vi "LLA_2_ECEF(SubVI).vi"(6 "f":dbl, 9 "alt(i) [m]":dbl, 10 "latd(i)":dbl, 11 "lon(i)":dbl) -> (3 "position":dbl[](array[numeric]))   [LabVIEW 2017]
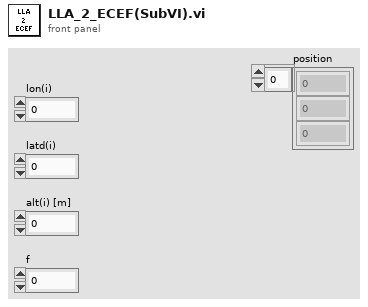
[diagram p1: front panel]
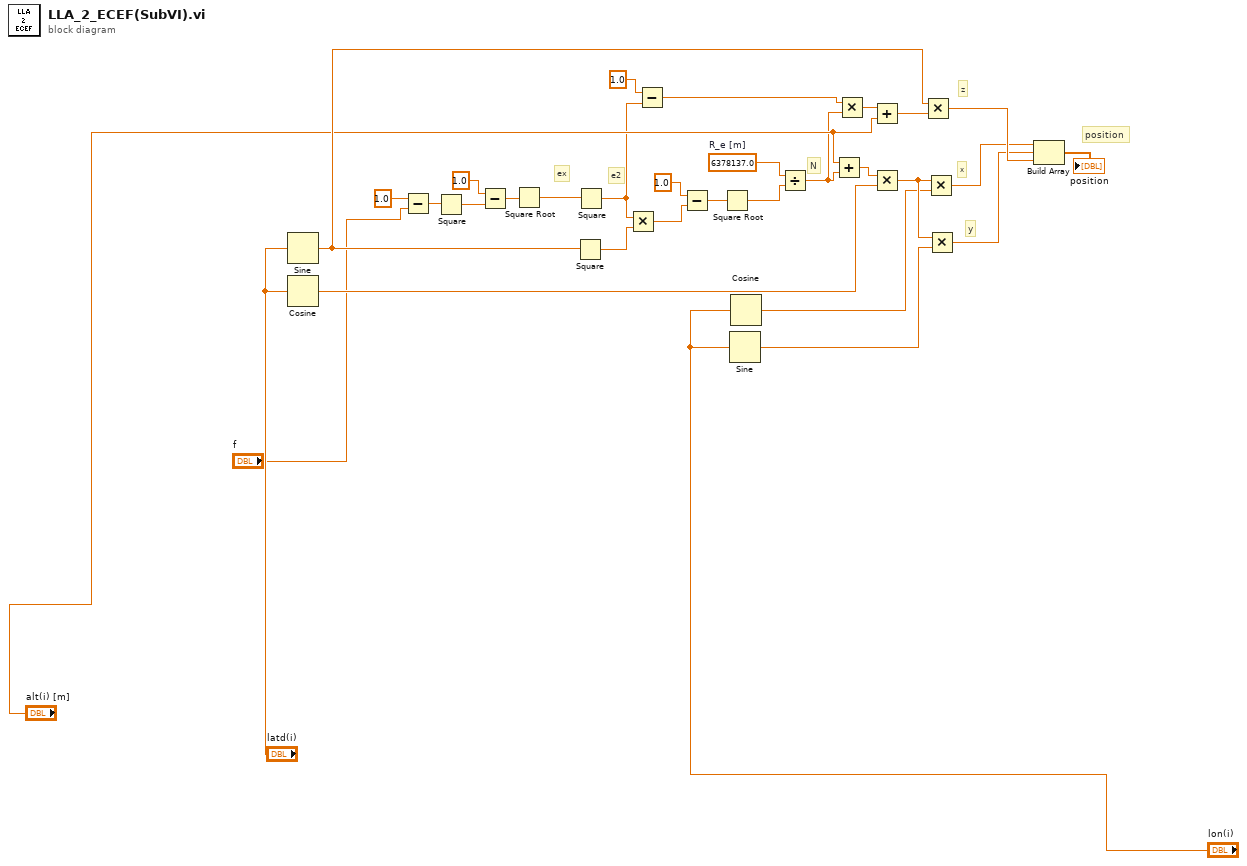
[diagram p0: block diagram]
diagram:
  w14 = 6378137.0  # R_e [m]
  # "position"
  # "z"
  # "y"
  # "x"
  # "N"
  # "e2"
  # "ex"
  n1 = Sine(x="latd(i)") -> (sin(x)=w29:dbl)
  n2 = Cosine(x="latd(i)") -> (cos(x)=w17:dbl)
  n3 = Subtract(x=1.0, y="f") -> (x-y=w6:dbl)
  n4 = Square(x=w6) -> (x^2=w7:dbl)
  n5 = Subtract(x=1.0, y=w7) -> (x-y=w5:dbl)
  n6 = Square Root(x=w5) -> (sqrt(x)=w9:dbl)
  n7 = Square(x=w29) -> (x^2=w10:dbl)
  n8 = Square(x=w9) -> (x^2=w23:dbl)
  n9 = Multiply(x=w23, y=w10) -> (x*y=w11:dbl)
  n10 = Subtract(x=1.0, y=w23) -> (x-y=w25:dbl)
  n11 = Subtract(x=1.0, y=w11) -> (x-y=w12:dbl)
  n12 = Square Root(x=w12) -> (sqrt(x)=w13:dbl)
  n13 = Sine(x="lon(i)") -> (sin(x)=w21:dbl)
  n14 = Cosine(x="lon(i)") -> (cos(x)=w18:dbl)
  n15 = Divide(x=w14, y=w13) -> (x/y=w24:dbl)
  n16 = Add(x="alt(i) [m]", y=w24) -> (x+y=w16:dbl)
  n17 = Multiply(x=w25, y=w24) -> (x*y=w26:dbl)
  n18 = Add(x=w26, y="alt(i) [m]") -> (x+y=w28:dbl)
  n19 = Multiply(x=w16, y=w17) -> (x*y=w20:dbl)
  n20 = Multiply(x=w29, y=w28) -> (x*y=w32:dbl)
  n21 = Multiply(x=w20, y=w18) -> (x*y=w30:dbl)
  n22 = Multiply(x=w20, y=w21) -> (x*y=w31:dbl)
  n23 = Build Array(w30, w31, w32) -> (→"position":dbl[])
